vi "write_itxFolder_to_cache.vi"(8 "error in (no error)":errorcluster, 10 "experiment folder (containing itx)":path, 11 "cache file path":path) -> (0 "error out":errorcluster, 1 "notes":string[](array[string]), 2 "wave names":string[](array[string]), 3 "written cache file out":path)   [LabVIEW 2016]
uses:
  <userlib>/_OpenG.lib/file/file.llb/Strip Path Extension - Path__ogtk.vi
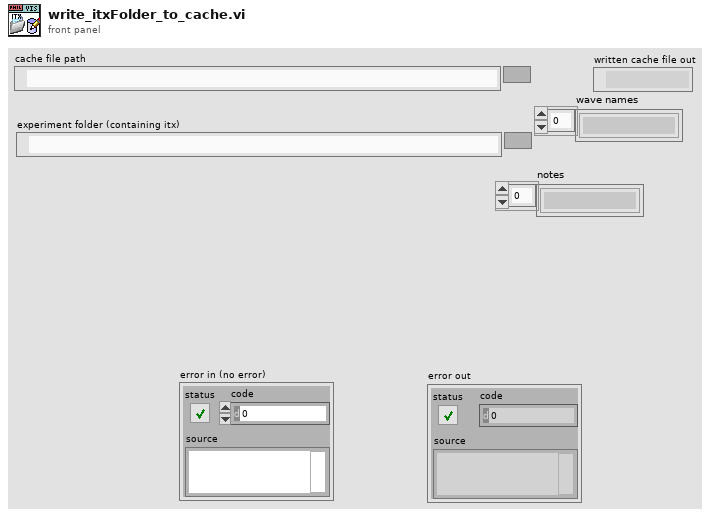
[diagram p1: front panel]
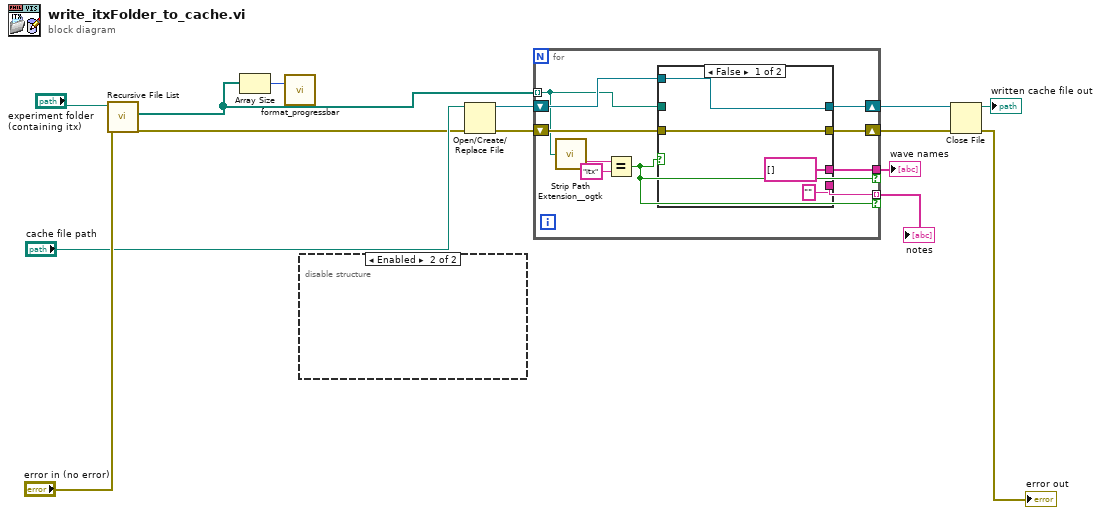
[diagram p0: block diagram]
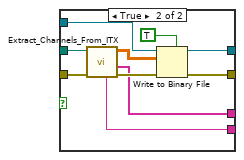
[diagram p3: hidden frame]
diagram:
  n1 = call <vilib>:"Recursive File List.vi"("error in (no error)"="error in (no error)", "Folder Path"="experiment folder (containing itx)") -> ("error out"=w4:errorcluster, "All Files in Dir"=w3:path[])  [unwired: 5 in, 3 out]
  n2 = Array Size(array=w3) -> (size(s)=w13:i32)
  n3 = call "format_progressbar.vi"("# itx files"=w13) -> ()  [unwired: 2 in, 1 out]
  n4 = disable-structure shown="Enabled" {
    frame Disabled {
    }
    frame Enabled {
    }
  }
  n5 = Open/Create/Replace File(file path (use dialog)="cache file path", error in=w4) -> (refnum out=w8:refnum<file>, error out=w11:errorcluster)  [unwired: 4 in, 1 out]
  n6 = for {
    tunnel: w3 -> [w18] mode=indexing
    shift-right: [w24] -> w5
    shift-left: w11 -> [w21]
    shift-right: [w23] -> w9
    shift-left: w8 -> [w22]
    tunnel: [w20] -> w2 mode=indexing if=w15
    tunnel: [w19] -> w1 if=w15
    n7 = call-poly <userlib>:"Strip Path Extension__ogtk.vi"("path"=w18) -> ("extension"=w17:string)  [unwired: 1 out]
    n8 = Equal?(x=w17, y="itx") -> (x = y?=w15:bool)
    n9 = case shown="False" w15 {
      tunnel: [w27 w35] -> w24
      tunnel: [w28 w34] -> w23
      tunnel: w22 -> [w28 w33]
      tunnel: w21 -> [w27 w32]
      tunnel: ["" ("Notes") w31] -> w20
      tunnel: [string[] [] ("wave names") w30] -> w19
      tunnel: w18 -> [_ w29]
      frame False {
      }
      frame True {
        n10 = call "Extract_Channels_From_ITX.vi"("error in"=w32, "itx file, N 1d channels"=w29) -> ("error out"=w36:errorcluster, "wave names"=w30:string[], "Arr of 1D channels"=w37:dbl[][], "Notes"=w31:string)  [unwired: 5 in, 1 out]
        n11 = Write to Binary File(file (use dialog)=w33, data=w37, error in=w36, 5:TRUE ("prepend array or string size? (T)")) -> (refnum out=w34:refnum<file>, error out=w35:errorcluster)  [unwired: 2 in, 1 out]
      }
    }
  }
  "notes" <- w2
  "wave names" <- w1
  n12 = Close File(refnum=w9, error in=w5) -> (path=→"written cache file out":path, error out=→"error out":errorcluster)
